vi "create_queue_volt.vi"(11 "Value":dbl) -> (2 "Current Queue":dbl[](array[numeric]), 3 "isEmpty":bool)   [LabVIEW 2016]
uses:
  <vilib>/ptbypt/NI_PtbyPt.lvlib
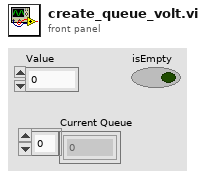
[diagram p1: front panel]
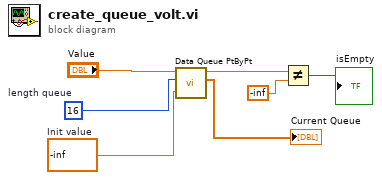
[diagram p0: block diagram]
diagram:
  w4 = -inf  # Init value
  w3 = 16  # length queue
  n1 = call <vilib>:"Data Queue PtByPt.vi"("initial queue element"=w4, "sample length"=w3, "input data point"="Value") -> ("Current Queue"=→"Current Queue":dbl[], "eliminated element"=w1:dbl)  [unwired: 4 in, 3 out]
  n2 = Not Equal?(x=w1, y=-inf) -> (x != y?=→"isEmpty":bool)
